vi "Split Function Select.vi"(0 "SYS.SELECT":u64 format="%.0x") -> (2 "Selector 1:0":fxp<+,4,4>, 3 "Selector 3:2":fxp<+,4,4>, 4 "Selector 7:4":fxp<+,8,8>, 6 "Selector 9:8":fxp<+,4,4>, 8 "Selector 11:10":fxp<+,4,4>, 10 "Selector 13:12":fxp<+,4,4>, 13 "Selector 19:18":fxp<+,4,4>, 14 "Selector 17:16":fxp<+,4,4>, 15 "Selector 15:14":fxp<+,4,4>)   [LabVIEW 2019]
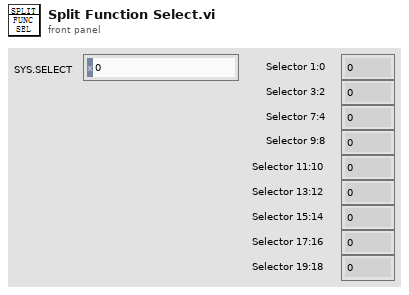
[diagram p1: front panel]
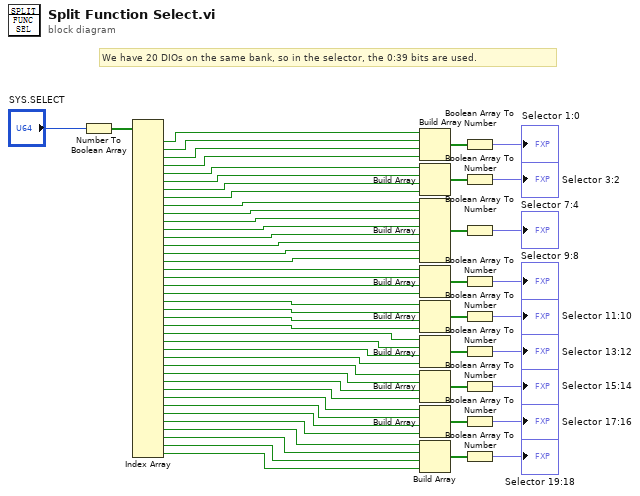
[diagram p0: block diagram]
diagram:
  # "We have 20 DIOs on the same bank, so in the selector, the 0:39 bits are used."
  n1 = Number To Boolean Array(number="SYS.SELECT") -> (Boolean array=w59:bool[])
  n2 = Index Array(array=w59) -> (element #1=w58:bool, element #2=w57:bool, element #3=w56:bool, element #4=w55:bool, element #5=w54:bool, element #6=w53:bool, element #7=w52:bool, element #8=w51:bool, element #9=w50:bool, element #10=w49:bool, element #11=w48:bool, element #12=w47:bool, element #13=w46:bool, element #14=w45:bool, element #15=w44:bool, element #16=w43:bool, element #17=w42:bool, element #18=w41:bool, element #19=w40:bool, element #20=w39:bool, element #21=w38:bool, element #22=w37:bool, element #23=w36:bool, element #24=w35:bool, element #25=w34:bool, element #26=w33:bool, element #27=w32:bool, element #28=w31:bool, element #29=w30:bool, element #30=w29:bool, element #31=w28:bool, element #32=w27:bool, element #33=w26:bool, element #34=w25:bool, element #35=w24:bool, element #36=w23:bool, element #37=w22:bool, element #38=w21:bool, element #39=w20:bool, element #40=w19:bool)  [unwired: 40 in]
  n3 = Build Array(w58, w57, w56, w55) -> (w18:bool[])
  n4 = Build Array(w54, w53, w52, w51) -> (w16:bool[])
  n5 = Build Array(w50, w49, w48, w47, w46, w45, w44, w43) -> (w15:bool[])
  n6 = Build Array(w42, w41, w40, w39) -> (w14:bool[])
  n7 = Build Array(w38, w37, w36, w35) -> (w13:bool[])
  n8 = Build Array(w34, w33, w32, w31) -> (w12:bool[])
  n9 = Build Array(w30, w29, w28, w27) -> (w11:bool[])
  n10 = Build Array(w26, w25, w24, w23) -> (w10:bool[])
  n11 = Build Array(w22, w21, w20, w19) -> (w9:bool[])
  n12 = Boolean Array To Number(Boolean array=w18) -> (number=→"Selector 1:0":fxp<+,4,4>)
  n13 = Boolean Array To Number(Boolean array=w16) -> (number=→"Selector 3:2":fxp<+,4,4>)
  n14 = Boolean Array To Number(Boolean array=w15) -> (number=→"Selector 7:4":fxp<+,8,8>)
  n15 = Boolean Array To Number(Boolean array=w14) -> (number=→"Selector 9:8":fxp<+,4,4>)
  n16 = Boolean Array To Number(Boolean array=w13) -> (number=→"Selector 11:10":fxp<+,4,4>)
  n17 = Boolean Array To Number(Boolean array=w12) -> (number=→"Selector 13:12":fxp<+,4,4>)
  n18 = Boolean Array To Number(Boolean array=w11) -> (number=→"Selector 15:14":fxp<+,4,4>)
  n19 = Boolean Array To Number(Boolean array=w10) -> (number=→"Selector 17:16":fxp<+,4,4>)
  n20 = Boolean Array To Number(Boolean array=w9) -> (number=→"Selector 19:18":fxp<+,4,4>)
